vi "GetSettingsFromDatabase.vi"() -> ()   [LabVIEW 2020]
uses:
  PXIController/settingsmanagement/DataBaseInterface/Controls/DataBaseOptions.ctl
  PXIController/settingsmanagement/DataBaseInterface/Controls/DataBaseAuthentication.ctl
  <vilib>/SAPHIR/GDataBase for MySQL(tm)/MySQL/MySQLConnector.lvclass/MySQLConnector.ctl
  <vilib>/SAPHIR/GDataBase for MySQL(tm)/NetworkStream/MySQLNetworkStream.lvclass/MySQLNetworkStream.ctl
  PXIController/settingsmanagement/DataBaseInterface/Private/GetMySQL_RT_Object.vi
  <vilib>/SAPHIR/GDataBase for MySQL(tm)/NetworkStream/public/SendCommand.vi
  <vilib>/SAPHIR/GDataBase for MySQL(tm)/NetworkStream/public/locker/AcquireLocker.vi
  <vilib>/SAPHIR/GDataBase for MySQL(tm)/NetworkStream/public/locker/ReleaseLocker.vi
  <vilib>/SAPHIR/GDataBase for MySQL(tm)/NetworkStream/public/WritePacket.vi
  <vilib>/SAPHIR/GDataBase for MySQL(tm)/MySQL/public/Open.vi
  <vilib>/Utility/error.llb/Trim Whitespace.vi
  <vilib>/Utility/semaphor.llb/Acquire Semaphore.vi
  <vilib>/SAPHIR/GDataBase for MySQL(tm)/NetworkStream/public/ReadResultPacket.vi
  <vilib>/Utility/semaphor.llb/Release Semaphore.vi
  <userlib>/_OpenG.lib/array/array.llb/Remove Duplicates from 1D Array (String)__ogtk.vi
  <vilib>/SAPHIR/GDataBase for MySQL(tm)/MySQL/MySQLConnector.lvclass
  PXIController/settingsmanagement/DataBaseInterface/DataBaseInterface.lvlib
panel:
  out "String":string
  out "error out":errorcluster
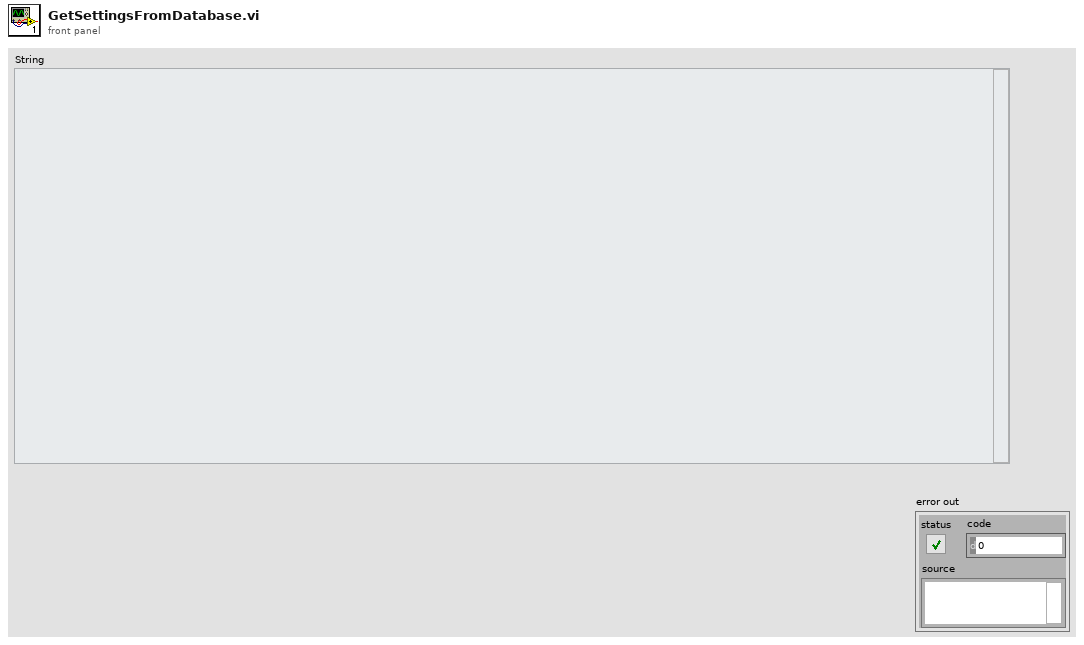
[diagram p1: front panel]
types:
  T1 = typedef "DataBaseInterface.lvlib/DataBaseAuthentication.ctl" = cluster{"username":string, "password":string, "database":string}
  T2 = typedef "DataBaseInterface.lvlib/DataBaseOptions.ctl" = cluster{"Timeout":u32, "Read Timeout":u32, "Auto Reconnect":bool}
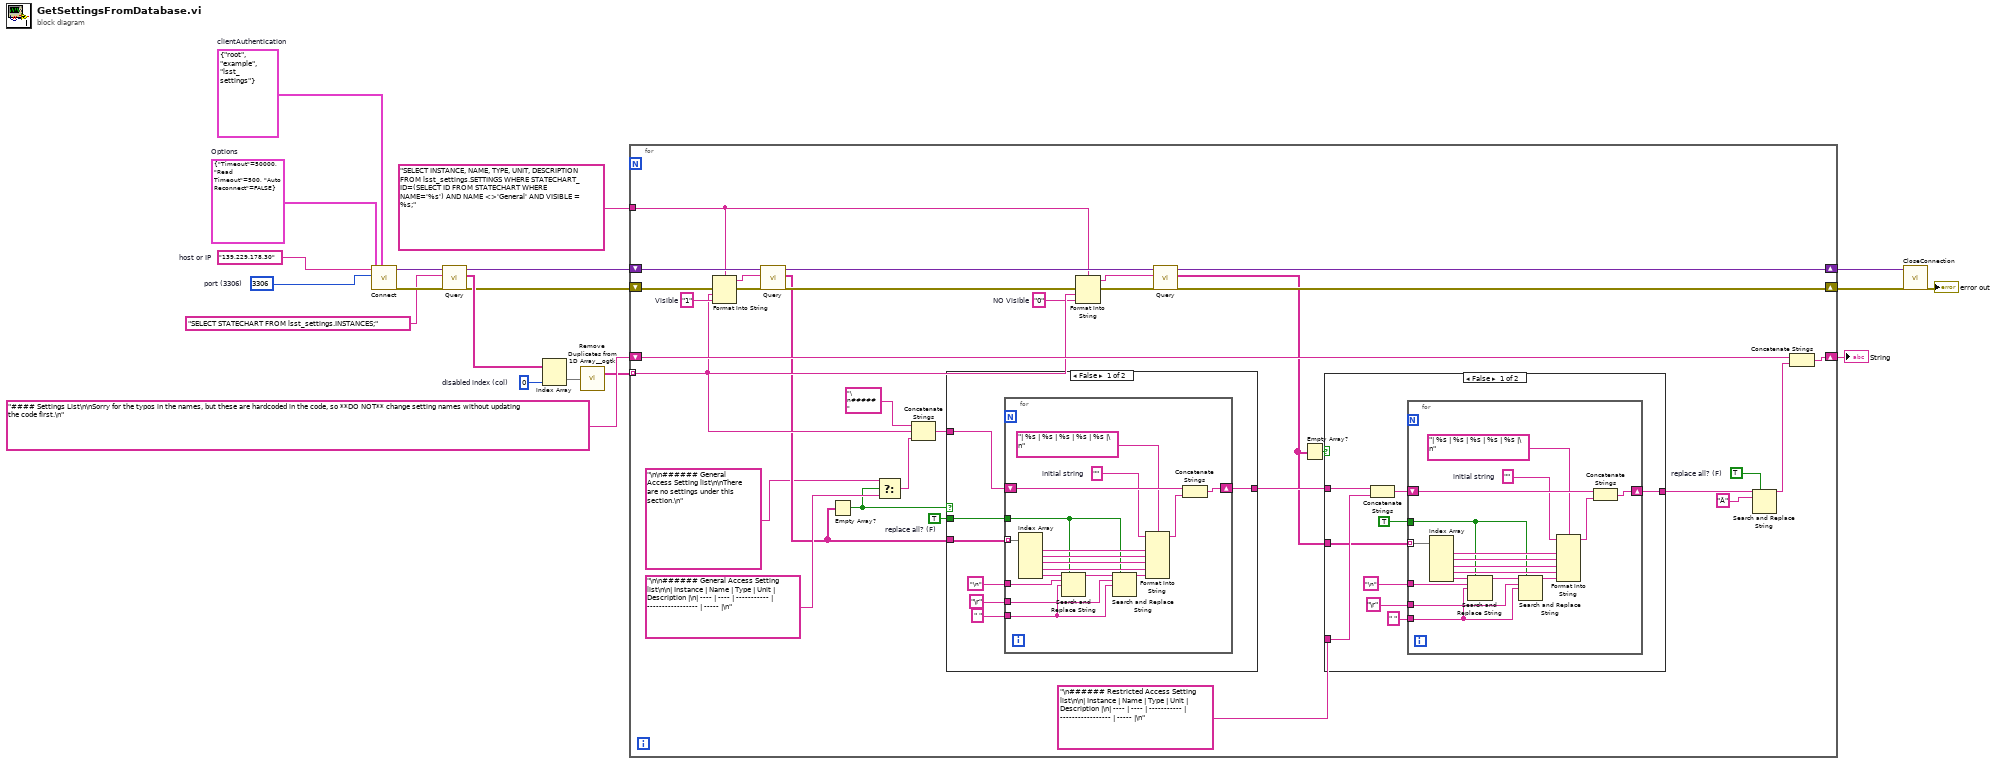
[diagram p0: block diagram]
diagram:
  w8 = 0  # disabled index (col)
  w13 = u16 3306  # port (3306)
  w14 = T1 {"username"="root", "password"="example", "database"="lsst_settings"}  # clientAuthentication
  w15 = T2 {"Timeout"=50000, "Read Timeout"=500, "Auto Reconnect"=FALSE}  # Options
  w16 = "139.229.178.30"  # host or IP
  n1 = call "Connect.vi"("clientAuthentication"=w14, "Options"=w15, "port (3306)"=w13, "host or IP"=w16) -> ("error out"=w18:errorcluster, "DatabaseObject out"=w19:variant)  [unwired: 6 in]
  n2 = call <vilib>:"Query.vi"("error in (no error)"=w18, "Query In"="SELECT STATECHART FROM lsst_settings.INSTANCES;", "DataBase Object"=w19) -> ("error out"=w4:errorcluster, "Query Results out"=w9:string[][], "DataBase Object out"=w5:variant)  [unwired: 6 in]
  n3 = Index Array(array=w9, index (col)=w8) -> (element=w7:string[])  [unwired: 1 in]
  n4 = call-poly <userlib>:"Remove Duplicates from 1D Array__ogtk.vi"("Input Array"=w7) -> ("Output Array"=w3:string[])  [unwired: 1 out]
  n5 = for {
    shift-right: [w50] -> w11
    shift-left: "#### Settings List\n\nSorry for the typos in the names, but these are hardcoded in the code, so **DO NOT** change setting names without updating the code first.\n" -> [w51]
    shift-right: [w32] -> w6
    shift-left: w5 -> [w49]
    shift-right: [w33] -> w1
    shift-left: w4 -> [w48]
    tunnel: w3 -> [w38] mode=indexing
    tunnel: "SELECT INSTANCE, NAME, TYPE, UNIT, DESCRIPTION FROM lsst_settings.SETTINGS WHERE STATECHART_ID=(SELECT ID FROM STATECHART WHERE NAME='%s') AND NAME <>'General' AND VISIBLE = %s;" -> [w36]
    w25 = TRUE  # replace all? (F)
    w29 = TRUE  # replace all? (F)
    w39 = "1"  # Visible
    w37 = "0"  # NO Visible
    n6 = Format Into String(format string=w36, error in=w48, w38, w39) -> (resulting string=w46:string, error out=w47:errorcluster)  [unwired: 1 in]
    n7 = call <vilib>:"Query.vi"("error in (no error)"=w47, "Query In"=w46, "DataBase Object"=w49) -> ("error out"=w40:errorcluster, "Query Results out"=w23:string[][], "DataBase Object out"=w41:variant)  [unwired: 6 in]
    n8 = Empty Array?(array=w23) -> (empty?=w21:bool)
    n9 = Select(t="\n\n###### General Access Setting list\n\nThere are no settings under this section.\n", s=w21, f="\n\n###### General Access Setting list\n\n| Instance | Name | Type | Unit | Description |\n| ---- | ---- | ----------- | ----------------- | ----- |\n") -> (s? t:f=w22:string)
    n10 = Concatenate Strings("\n##### ", w38, w22) -> (w24:string)
    n11 = case shown="False" w21 {
      tunnel: w23 -> [w58 _]
      tunnel: w24 -> [w57 w76]
      tunnel: [w56 w76] -> w43
      tunnel: w29 -> [w55 _]
      frame False {
        n12 = for {
          tunnel: w58 -> [w67] mode=indexing
          shift-right: [w66] -> w56
          shift-left: w57 -> [w75]
          tunnel: w55 -> [w61]
          tunnel: "\n" -> [w64]
          tunnel: " " -> [w60]
          tunnel: "\r" -> [w59]
          w73 = ""  # initial string
          n13 = Index Array(array=w67) -> (element #1=w68:string, element #2=w72:string, element #3=w71:string, element #4=w70:string, element #5=w69:string)  [unwired: 5 in]
          n14 = Search and Replace String(replace all?=w61, input string=w69, search string=w64, replace string=w60) -> (result string=w63:string)  [unwired: 4 in, 3 out]
          n15 = Search and Replace String(replace all?=w61, input string=w63, search string=w59, replace string=w60) -> (result string=w62:string)  [unwired: 4 in, 3 out]
          n16 = Format Into String(format string="| %s | %s | %s | %s | %s |\n", initial string=w73, w68, w72, w71, w70, w62) -> (resulting string=w65:string)  [unwired: 1 in, 1 out]
          n17 = Concatenate Strings(w75, w65) -> (w66:string)
        }
      }
      frame True {
      }
    }
    n18 = Format Into String(format string=w36, error in=w40, w38, w37) -> (resulting string=w35:string, error out=w34:errorcluster)  [unwired: 1 in]
    n19 = call <vilib>:"Query.vi"("error in (no error)"=w34, "Query In"=w35, "DataBase Object"=w41) -> ("error out"=w33:errorcluster, "Query Results out"=w31:string[][], "DataBase Object out"=w32:variant)  [unwired: 6 in]
    n20 = Empty Array?(array=w31) -> (empty?=w30:bool)
    n21 = case shown="False" w30 {
      tunnel: w43 -> [w85 w103]
      tunnel: "\n###### Restricted Access Setting list\n\n| Instance | Name | Type | Unit | Description |\n| ---- | ---- | ----------- | ----------------- | ----- |\n" -> [w84 _]
      tunnel: [w82 w103] -> w28
      tunnel: w31 -> [w81 _]
      frame False {
        n22 = Concatenate Strings(w85, w84) -> (w83:string)
        n23 = for {
          tunnel: w81 -> [w95] mode=indexing
          shift-right: [w94] -> w82
          shift-left: w83 -> [w102]
          tunnel: TRUE -> [w89]
          tunnel: "\n" -> [w88]
          tunnel: "\r" -> [w87]
          tunnel: " " -> [w86]
          w100 = ""  # initial string
          n24 = Index Array(array=w95) -> (element #1=w96:string, element #2=w99:string, element #3=w98:string, element #4=w97:string, element #5=w92:string)  [unwired: 5 in]
          n25 = Search and Replace String(replace all?=w89, input string=w92, search string=w88, replace string=w86) -> (result string=w91:string)  [unwired: 4 in, 3 out]
          n26 = Search and Replace String(replace all?=w89, input string=w91, search string=w87, replace string=w86) -> (result string=w90:string)  [unwired: 4 in, 3 out]
          n27 = Format Into String(format string="| %s | %s | %s | %s | %s |\n", initial string=w100, w96, w99, w98, w97, w90) -> (resulting string=w93:string)  [unwired: 1 in, 1 out]
          n28 = Concatenate Strings(w102, w93) -> (w94:string)
        }
      }
      frame True {
      }
    }
    n29 = Search and Replace String(replace all?=w25, input string=w28, search string="Â") -> (result string=w26:string)  [unwired: 5 in, 3 out]
    n30 = Concatenate Strings(w51, w26) -> (w50:string)
  }
  "String" <- w11
  n31 = call "CloseConnection.vi"("error in (no error)"=w1, "DataBase Object"=w6) -> ("error out"=→"error out":errorcluster)  [unwired: 9 in]
